vi "InitCam3030.vi"(7 "error in (no error)":errorcluster) -> (0 "error out":errorcluster)   [LabVIEW 2015, in "ESLSCDLL.lvlib"]
uses:
  ESLSCDLL.lvlib
  Globals.vi
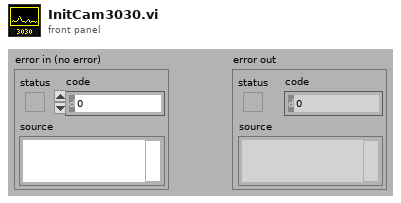
[diagram p1: front panel]
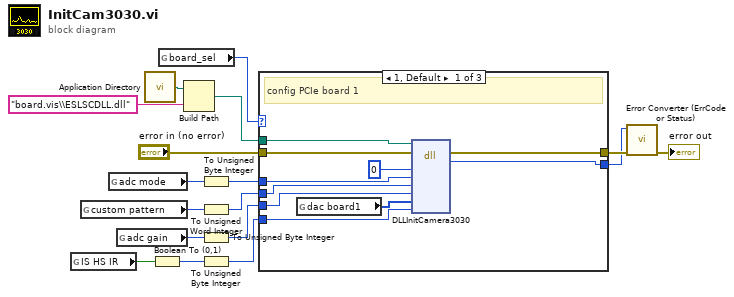
[diagram p0: block diagram]
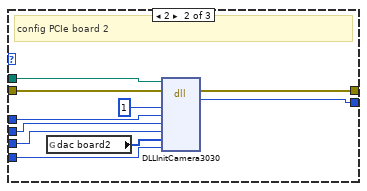
[diagram p2: hidden frame]
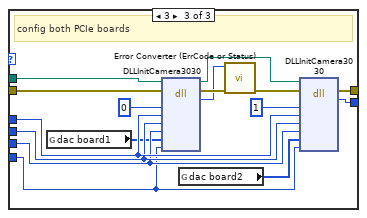
[diagram p3: hidden frame]
diagram:
  n1 = global read "Globals.vi" "IS HS IR"() -> (w6:bool)
  n2 = global read "Globals.vi" "custom pattern"() -> (w10:u32)
  n3 = global read "Globals.vi" "adc mode"() -> (w9:enum16{"normal", "ramp", "custom pattern"})
  n4 = global read "Globals.vi" "adc gain"() -> (w12:u32)
  n5 = call <vilib>:"Application Directory.vi"() -> ("Application Directory"=w3:path)
  n6 = Boolean To (0,1)(Boolean=w6) -> (0, 1=w5:i16)
  n7 = global read "Globals.vi" "board_sel"() -> (w13:u32)
  n8 = Build Path(base path=w3, name or relative path="board.vis\\ESLSCDLL.dll") -> (appended path=w1:path)
  n9 = To Unsigned Byte Integer(number=w9) -> (unsigned 8bit integer=w8:u8)
  n10 = To Unsigned Word Integer(number=w10) -> (unsigned 16bit integer=w7:u16)
  n11 = To Unsigned Byte Integer(number=w12) -> (unsigned 8bit integer=w11:u8)
  n12 = To Unsigned Byte Integer(number=w5) -> (unsigned 8bit integer=w4:u8)
  n13 = case shown="1, Default" w13 {
    tunnel: w8 -> [w27 w36 w47]
    tunnel: w7 -> [w26 w35 w46]
    tunnel: w11 -> [w25 w34 w45]
    tunnel: "error in (no error)" -> [w24 w37 w53]
    tunnel: [w23 w32 w44] -> w16
    tunnel: [w22 w33 w43] -> w14
    tunnel: w4 -> [w21 w31 w42]
    tunnel: w1 -> [w19 w29 w39]
    frame 1, Default {
      # "config PCIe board 1"
      n14 = global read "Globals.vi" "dac board1"() -> (w20:u32[])
      n15 = dll-call lib="C:/ENTW/PCIE/LV64/board.vis/ESLSCDLL.dll" fn="DLLInitCamera3030" ("lwlscdll.dll:DLLWriteLongS0")(path in=w19, error in=w24, "drvno"=u32 0, "adc_mode"=w27, "custom_pattern"=w26, "adc_gain"=w25, "dac_output"=w20, "isIR"=w21) -> (error out=w23:errorcluster, "es_status_codes"=w22:i32)  [unwired: 7 in, 1 out]
    }
    frame 2 {
      # "config PCIe board 2"
      n16 = global read "Globals.vi" "dac board2"() -> (w30:u32[])
      n17 = dll-call lib="C:/ENTW/PCIE/LV64/board.vis/ESLSCDLL.dll" fn="DLLInitCamera3030" ("lwlscdll.dll:DLLWriteLongS0")(path in=w29, error in=w37, "drvno"=u32 1, "adc_mode"=w36, "custom_pattern"=w35, "adc_gain"=w34, "dac_output"=w30, "isIR"=w31) -> (error out=w32:errorcluster, "es_status_codes"=w33:i32)  [unwired: 7 in, 1 out]
    }
    frame 3 {
      # "config both PCIe boards"
      n18 = global read "Globals.vi" "dac board1"() -> (w41:u32[])
      n19 = dll-call lib="C:/ENTW/PCIE/LV64/board.vis/ESLSCDLL.dll" fn="DLLInitCamera3030" ("lwlscdll.dll:DLLWriteLongS0")(path in=w39, error in=w53, "drvno"=u32 0, "adc_mode"=w47, "custom_pattern"=w46, "adc_gain"=w45, "dac_output"=w41, "isIR"=w42) -> (path out=w38:path, error out=w51:errorcluster, "es_status_codes"=w50:i32)  [unwired: 7 in]
      n20 = global read "Globals.vi" "dac board2"() -> (w40:u32[])
      n21 = call "Error Converter (ErrCode or Status).vi"("error in (no error)"=w51, "error code"=w50) -> ("error out"=w49:errorcluster)  [unwired: 9 in]
      n22 = dll-call lib="C:/ENTW/PCIE/LV64/board.vis/ESLSCDLL.dll" fn="DLLInitCamera3030" ("lwlscdll.dll:DLLWriteLongS0")(path in=w38, error in=w49, "drvno"=u32 1, "adc_mode"=w47, "custom_pattern"=w46, "adc_gain"=w45, "dac_output"=w40, "isIR"=w42) -> (error out=w44:errorcluster, "es_status_codes"=w43:i32)  [unwired: 7 in, 1 out]
    }
  }
  n23 = call "Error Converter (ErrCode or Status).vi"("error in (no error)"=w16, "error code"=w14) -> ("error out"=→"error out":errorcluster)  [unwired: 9 in]
